vi "5056_60_set_single_output.vi"(0 "Channel Name":string, 1 "Address (all reqd.)":T1, 2 "Set state:":bool) -> (3 "Comment":string, 6 "Good Reply":bool)   [LabVIEW 2010]
uses:
  ADAM Client/Sub VIs/ADAM Controls/Address.ctl
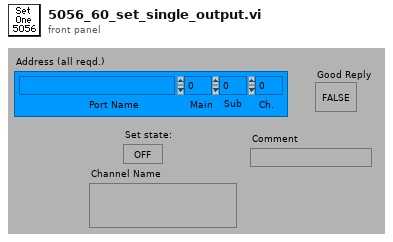
[diagram p1: front panel]
types:
  T1 = typedef "Address.ctl" = cluster{"Main":i32, "Ch.":i32, "Sub":i32, "Port Name":string}
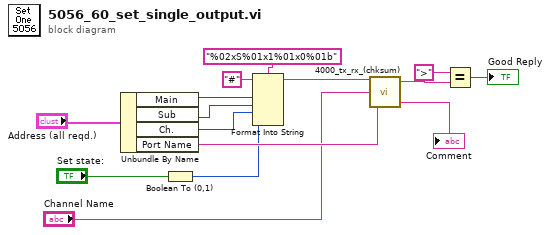
[diagram p0: block diagram]
diagram:
  n1 = Unbundle By Name("Address (all reqd.)") -> ("Main"=w14:i32, "Sub"=w15:i32, "Ch."=w7:i32, "Port Name"=w8:string)
  n2 = Boolean To (0,1)(Boolean="Set state:") -> (0, 1=w2:i16)
  n3 = Format Into String(format string="%02xS%01x1%01x0%01b", initial string="#", w14, w15, w7, w2) -> (resulting string=w11:string)  [unwired: 1 in, 1 out]
  n4 = call "4000_tx_rx_(chksum).vi"("Port Name"=w8, "Channel Name"="Channel Name", "Write String"=w11) -> ("Comment out"=→"Comment":string, "Read"=w4:string)  [unwired: 1 out]
  n5 = Equal?(x=">", y=w4) -> (x = y?=→"Good Reply":bool)
